vi "GetOwnedClassList.vi"(8 "error in (no error)":errorcluster, 11 "Project Path":path=path "E:/sw-deps-monitor/Source/BuildSpecs/Modules/ModuleA.lvproj") -> (0 "error out":errorcluster, 3 "Owned Class[]":path[](array[path]))   [LabVIEW 2019, in "DepsWatch.lvlib"]
uses:
  DepsWatch.lvlib
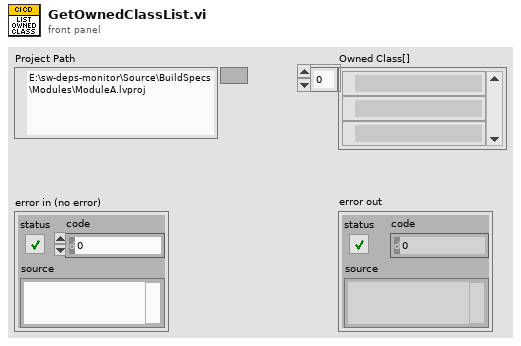
[diagram p1: front panel]
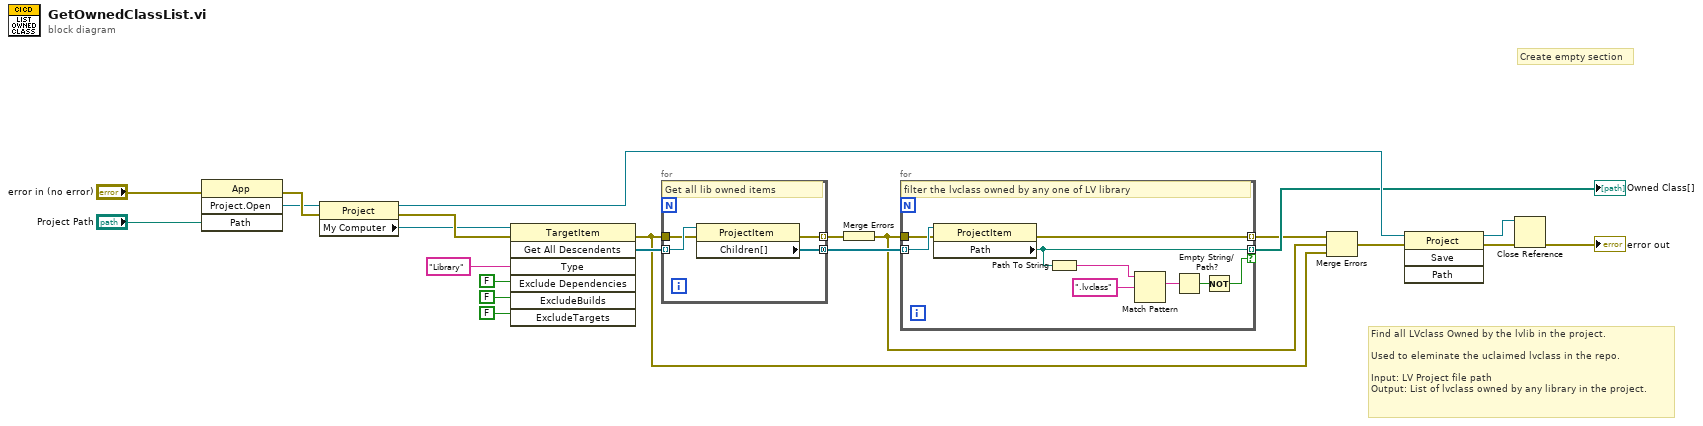
[diagram p0: block diagram]
diagram:
  # "Find all LVclass Owned by the lvlib in the project.\n\nUsed to eleminate the uclaimed lvclass in the repo.\n\nInput: LV Project file path\nOutput: List of lvclass owned by any library in the project."
  # "Create empty section"
  n1 = invoke class="App" method="Project.Open"(error in="error in (no error)", "Path"="Project Path") -> (error out=w21:errorcluster, "Project:Open"=w11:refnum<vi>)  [unwired: 2 in, 2 out]
  n2 = property class="Project"(reference=w11, error in=w21) -> (reference out=w16:refnum<vi>, error out=w17:errorcluster, "My Computer"=w10:refnum<vi>)
  n3 = invoke class="TargetItem" method="Get All Descendents"(reference=w10, error in=w17, "Type"="Library", "Exclude Dependencies"=FALSE ("ExcludeDependencies"), "ExcludeBuilds"=FALSE, "ExcludeTargets"=FALSE) -> (error out=w2:errorcluster, "All Descendents"=w9:refnum<vi>[])  [unwired: 1 in, 5 out]
  n4 = for {
    tunnel: w9 -> [w26] mode=indexing
    tunnel: [w25] -> w7 mode=concatenating
    tunnel: w2 -> [w24]
    tunnel: [w23] -> w5 mode=indexing
    # "Get all lib owned items"
    n5 = property class="ProjectItem"(reference=w26, error in=w24) -> (error out=w23:errorcluster, "Children[]"=w25:refnum<vi>[])  [unwired: 1 out]
  }
  n6 = Merge Errors(w5) -> (w1:errorcluster)
  n7 = for {
    tunnel: w7 -> [w35] mode=indexing
    tunnel: [w31] -> w6 mode=indexing if=w29
    tunnel: w1 -> [w28]
    tunnel: [w27] -> w4 mode=indexing
    # "filter the lvclass owned by any one of LV library"
    n8 = property class="ProjectItem"(reference=w35, error in=w28) -> (error out=w27:errorcluster, "Path"=w31:path)  [unwired: 1 out]
    n9 = Path To String(path=w31) -> (string=w34:string)
    n10 = Match Pattern(string=w34, regular expression=".lvclass") -> (match substring=w32:string)  [unwired: 1 in, 3 out]
    n11 = Empty String/Path?(string/path=w32) -> (empty?=w30:bool)
    n12 = Not(x=w30) -> (.not. x?=w29:bool)
  }
  "Owned Class[]" <- w6
  n13 = Merge Errors(w4, w1, w2) -> (w3:errorcluster)
  n14 = invoke class="Project" method="Save"(reference=w16, error in=w3) -> (reference out=w15:refnum<vi>, error out=w14:errorcluster)  [unwired: 2 in, 2 out]
  n15 = Close Reference(reference=w15, error in (no error)=w14) -> (error out=→"error out":errorcluster)
